vi "BackupRecipeFiles.vi"() -> ()   [LabVIEW 2012]
uses:
  <vilib>/addons/database/Connection.llb/DB Tools Open Connec (Path).vi
  <vilib>/addons/database/Connection.llb/Conn Execute.vi
  <vilib>/addons/database/Recordset.llb/Rec Fetch Recordset Data (R).vi
  <vilib>/addons/database/Recordset.llb/Rec Destroy - Connection.vi
  <vilib>/addons/database/_DB Variant To Data/Database Variant To Data.xnode
  <vilib>/addons/database/NI_Database_API.lvlib
panel:
  out "error out 2":errorcluster
  out "appended path 2":path
  out "appended path":path
  out "before substring 2":string
  out "error out":errorcluster
  out "before substring":string
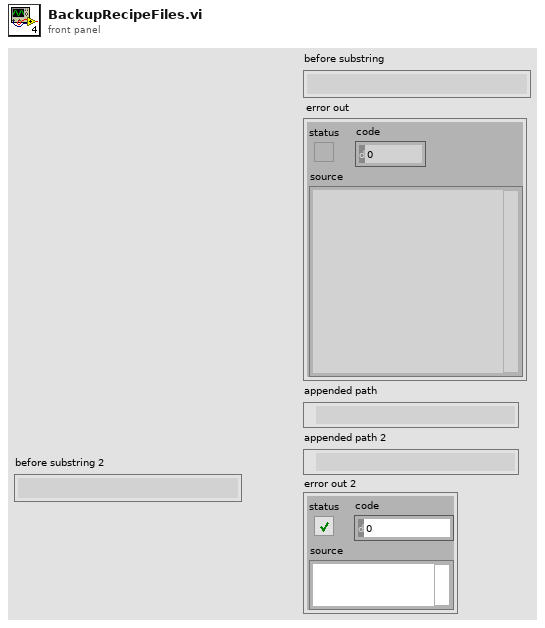
[diagram p1: front panel]
types:
  T1 = typedef "NI_Database_API.lvlib/Conn ObjectReference.ctl" = refnum<k1>
  T2 = typedef "NI_Database_API.lvlib/Rec ObjectReference.ctl" = refnum<k1>
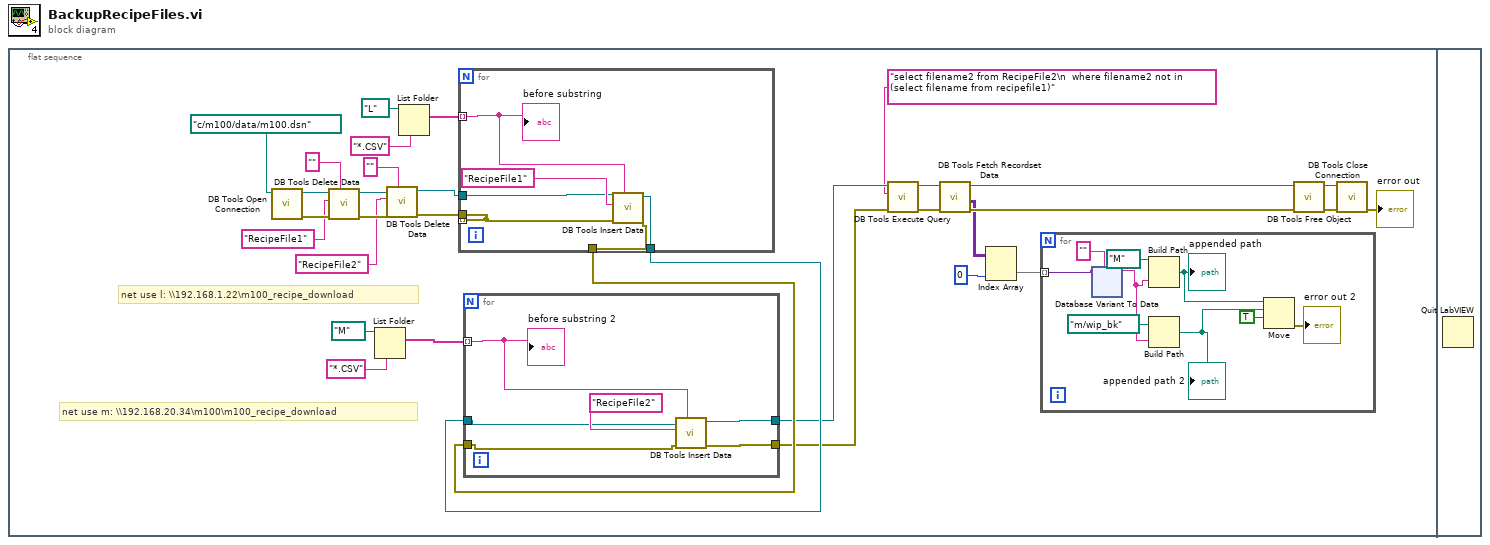
[diagram p0: block diagram]
diagram:
  n1 = flat-sequence {
    frame #0 {
      # "net use l: \\\\192.168.1.22\\m100_recipe_download"
      # "net use m: \\\\192.168.20.34\\m100\\m100_recipe_download"
      n2 = call-poly <vilib>:"DB Tools Open Connection.vi"("connection information"=path "c:/m100/data/m100.dsn") -> ("error out"=w22:errorcluster, "connection reference"=w21:T1)  [unwired: 7 in]
      n3 = call <vilib>:"DB Tools Delete Data.vi"("condition"="", "error in (no error)"=w22, "table"="RecipeFile1", "connection reference"=w21) -> ("error out"=w20:errorcluster, "connection reference out"=w19:T1)  [unwired: 6 in]
      n4 = List Folder(path=path "M:/", pattern="*.CSV") -> (filenames=w25:string[])  [unwired: 2 in, 3 out]
      n5 = call <vilib>:"DB Tools Delete Data.vi"("condition"="", "error in (no error)"=w20, "table"="RecipeFile2", "connection reference"=w19) -> ("error out"=w13:errorcluster, "connection reference out"=w14:T1)  [unwired: 6 in]
      n6 = List Folder(path=path "L:/", pattern="*.CSV") -> (filenames=w30:string[])  [unwired: 2 in, 3 out]
      n7 = for {
        tunnel: w30 -> [w85] mode=indexing
        tunnel: w14 -> [w81]
        tunnel: [w80] -> _ mode=indexing
        tunnel: [w84] -> w24
        tunnel: [w83] -> w23
        tunnel: w13 -> [w80]
        n8 = call <vilib>:"DB Tools Insert Data.vi"("data"=w85, "error in (no error)"=w80, "table"="RecipeFile1", "connection reference"=w81) -> ("error out"=w83:errorcluster, "connection reference out"=w84:T1)  [unwired: 6 in]
        "before substring" <- w85
      }
      n9 = for {
        tunnel: w25 -> [w77] mode=indexing
        tunnel: w24 -> [w75]
        tunnel: w23 -> [w74]
        tunnel: [w79] -> w6
        tunnel: [w78] -> w5
        n10 = call <vilib>:"DB Tools Insert Data.vi"("data"=w77, "error in (no error)"=w74, "table"="RecipeFile2", "connection reference"=w75) -> ("error out"=w78:errorcluster, "connection reference out"=w79:T1)  [unwired: 6 in]
        "before substring 2" <- w77
      }
      n11 = call-poly <vilib>:"DB Tools Execute Query.vi"("error in (no error)"=w5, "SQL query"="select filename2 from RecipeFile2\n  where filename2 not in (select filename from recipefile1)", "connection reference"=w6) -> ("error out"=w12:errorcluster, "recordset reference"=w11:T2)  [unwired: 5 in]
      n12 = call-poly <vilib>:"DB Tools Fetch Recordset Data.vi"("error in (no error)"=w12, "recordset reference"=w11) -> ("error out"=w9:errorcluster, "recordset data"=w3:variant[][], "recordset reference out"=w10:T2)  [unwired: 3 in]
      n13 = Index Array(array=w3, index (col)=0 ("disabled index (col)")) -> (element=w1:variant[])  [unwired: 1 in]
      n14 = for {
        tunnel: w1 -> [w41] mode=indexing
        n15 = xnode "Database Variant To Data"("database variant"=w41, "type"="") -> ("data"=w39:string)  [unwired: 1 in, 1 out]
        n16 = Build Path(base path=path "M:/", name or relative path=w39) -> (appended path=w36:path)
        "appended path" <- w36
        n17 = Build Path(base path=path "m:/wip_bk", name or relative path=w39) -> (appended path=w35:path)
        "appended path 2" <- w35
        n18 = Move(source path=w36, 9:TRUE ("overwrite (F)"), 10:w35) -> (error out=→"error out 2":errorcluster)  [unwired: 2 in, 2 out]
      }
      n19 = call-poly <vilib>:"DB Tools Free Object.vi"("error in (no error)"=w9, "recordset reference"=w10) -> ("error out"=w7:errorcluster, "connection reference"=w8:T1)  [unwired: 8 in]
      n20 = call <vilib>:"DB Tools Close Connection.vi"("error in (no error)"=w7, "connection reference"=w8) -> ("error out"=→"error out":errorcluster)  [unwired: 5 in]
    }
    frame #1 {
      n21 = Quit LabVIEW() -> ()  [unwired: 1 in]
    }
  }
